vi "Get Events.vi"(11 "Test Channel Charm View in":refnum<class "Test Channel Charm View.lvclass">) -> (2 "Events":T1, 3 "Test Channel Charm View out":refnum<class "Test Channel Charm View.lvclass">)   [LabVIEW 2013, in "Test Channel Charm View.lvlib" / "Test Channel Charm View.lvclass"]
uses:
  Test Channel Charm View.lvclass
  Typedef/Events.ctl
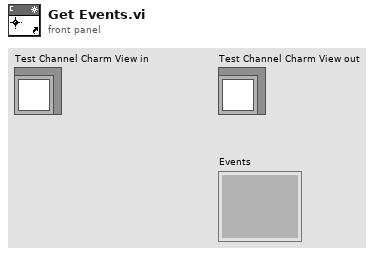
[diagram p1: front panel]
types:
  T1 = typedef "Test Channel Charm View.lvlib/Test Channel Charm View.lvclass/Events.ctl" = cluster{}
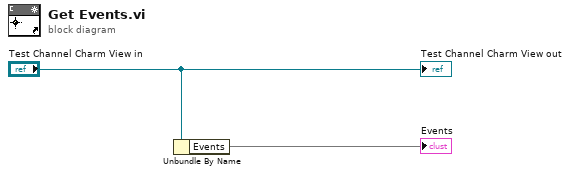
[diagram p0: block diagram]
diagram:
  n1 = Unbundle By Name("Test Channel Charm View in") -> ("Events"=→"Events")
  "Test Channel Charm View out" <- "Test Channel Charm View in"
